vi "convert_string2list.vi"(0 "PARSED STRING":string, 2 "BEGIN (CHAR)":string, 3 "TERM (CHAR)":string, 4 "CLUSTER (CHAR)":string, 5 "SEPARATOR (CHAR)":string) -> (14 "LIST":string[](array[string]), 19 "ERROR OUT":errorcluster)   [LabVIEW 2018, in "db_lib R3.lvlib"]
uses:
  db_lib R3.lvlib
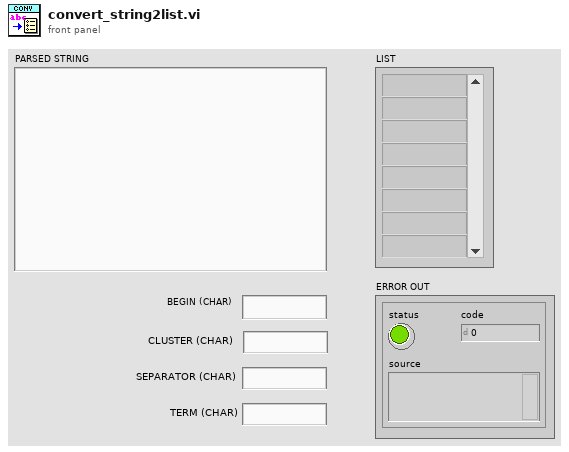
[diagram p1: front panel]
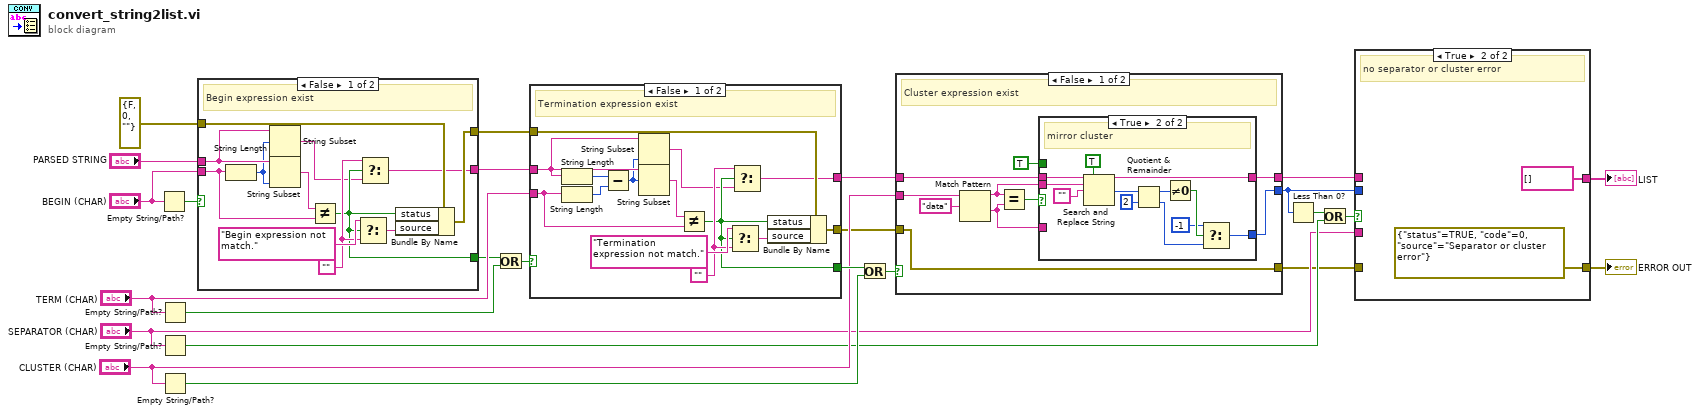
[diagram p0: block diagram]
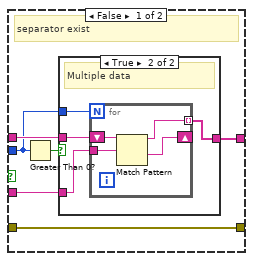
[diagram p2: hidden frame]
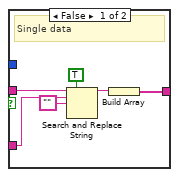
[diagram p3: hidden frame]
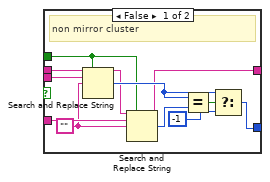
[diagram p4: hidden frame]
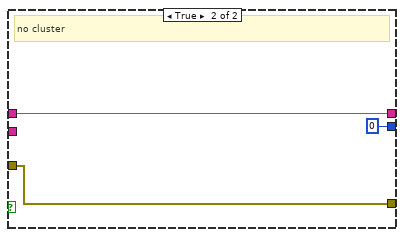
[diagram p5: hidden frame]
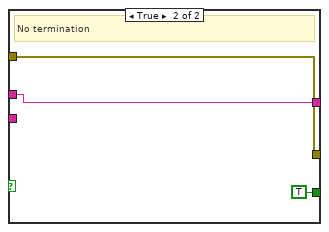
[diagram p6: hidden frame]
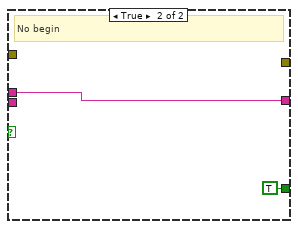
[diagram p7: hidden frame]
diagram:
  n1 = Empty String/Path?(string/path="BEGIN (CHAR)") -> (empty?=w25:bool)
  n2 = Empty String/Path?(string/path="TERM (CHAR)") -> (empty?=w16:bool)
  n3 = Empty String/Path?(string/path="SEPARATOR (CHAR)") -> (empty?=w7:bool)
  n4 = Empty String/Path?(string/path="CLUSTER (CHAR)") -> (empty?=w9:bool)
  n5 = case shown="False" w25 {
    tunnel: "PARSED STRING" -> [w34 w39]
    tunnel: [w30 w39] -> w21
    tunnel: "BEGIN (CHAR)" -> [w35 _]
    tunnel: errorcluster {"status"=FALSE, "code"=0, "source"=""} ("error constant") -> [w36 _]
    tunnel: [w31 _] -> w20
    tunnel: [w27 TRUE] -> w17
    frame False {
      w28 = ""
      # "Begin expression exist"
      n6 = String Length(string=w35) -> (length=w33:i32)
      n7 = String Subset(string=w34, offset (0)=w33) -> (substring=w26:string)  [unwired: 1 in]
      n8 = String Subset(string=w34, length (rest)=w33) -> (substring=w37:string)  [unwired: 1 in]
      n9 = Not Equal?(x=w37, y=w35) -> (x != y?=w27:bool)
      n10 = Select(t="Begin expression not match.", s=w27, f=w28) -> (s? t:f=w32:string)
      n11 = Select(t=w28, s=w27, f=w26) -> (s? t:f=w30:string)
      n12 = Bundle By Name(cluster=w36, "status"=w27, "source"=w32) -> (w31:errorcluster)
    }
    frame True {
      # "No begin"
    }
  }
  n13 = Or(x=w17, y=w16) -> (x .or. y?=w19:bool)
  n14 = case shown="False" w19 {
    tunnel: w21 -> [w46 w54]
    tunnel: [w49 w54] -> w14
    tunnel: "TERM (CHAR)" -> [w52 _]
    tunnel: w20 -> [w53 w56]
    tunnel: [w50 w56] -> w11
    tunnel: [w41 TRUE] -> w15
    frame False {
      w47 = ""
      # "Termination expression exist"
      n15 = String Length(string=w46) -> (length=w45:i32)
      n16 = String Length(string=w52) -> (length=w44:i32)
      n17 = Subtract(x=w45, y=w44) -> (x-y=w42:i32)
      n18 = String Subset(string=w46, length (rest)=w42) -> (substring=w40:string)  [unwired: 1 in]
      n19 = String Subset(string=w46, offset (0)=w42) -> (substring=w43:string)  [unwired: 1 in]
      n20 = Not Equal?(x=w43, y=w52) -> (x != y?=w41:bool)
      n21 = Select(t="Termination expression not match.", s=w41, f=w47) -> (s? t:f=w51:string)
      n22 = Select(t=w47, s=w41, f=w40) -> (s? t:f=w49:string)
      n23 = Bundle By Name(cluster=w53, "status"=w41, "source"=w51) -> (w50:errorcluster)
    }
    frame True {
      # "No termination"
    }
  }
  n24 = Or(x=w15, y=w9) -> (x .or. y?=w13:bool)
  n25 = case shown="False" w13 {
    tunnel: w14 -> [w63 w93]
    tunnel: "CLUSTER (CHAR)" -> [w66 _]
    tunnel: [w59 w93] -> w6
    tunnel: [w58 0 ("t")] -> w4
    tunnel: w11 -> [w57 w91]
    tunnel: [w57 w91] -> w2
    frame False {
      # "Cluster expression exist"
      n26 = Match Pattern(string=w66, regular expression="data") -> (before substring=w62:string, after substring=w61:string)  [unwired: 1 in, 2 out]
      n27 = Equal?(x=w62, y=w61) -> (x = y?=w64:bool)
      n28 = case shown="True" w64 {
        tunnel: w63 -> [w77 w90]
        tunnel: w62 -> [w78 w89]
        tunnel: [w68 w86] -> w59
        tunnel: w61 -> [w76 _]
        tunnel: [w71 w79] -> w58
        tunnel: TRUE -> [w67 _]
        frame False {
          w70 = ""
          # "non mirror cluster"
          n29 = Search and Replace String(replace all?=w67, input string=w77, search string=w78, replace string=w70) -> (result string=w69:string, number of replacements=w73:i32)  [unwired: 4 in, 2 out]
          n30 = Search and Replace String(replace all?=w67, input string=w69, search string=w76, replace string=w70) -> (result string=w68:string, number of replacements=w74:i32)  [unwired: 4 in, 2 out]
          n31 = Equal?(x=w73, y=w74) -> (x = y?=w75:bool)
          n32 = Select(t=w73, s=w75, f=-1) -> (s? t:f=w71:i32)
        }
        frame True {
          # "mirror cluster"
          n33 = Search and Replace String(replace all?=TRUE ("replace all? (F)"), input string=w90, search string=w89, replace string="") -> (result string=w86:string, number of replacements=w85:i32)  [unwired: 4 in, 2 out]
          n34 = Quotient & Remainder(x=w85, y=2) -> (x-y*floor(x/y)=w84:i32, floor(x/y)=w82:i32)
          n35 = Not Equal To 0?(x=w84) -> (x != 0?=w83:bool)
          n36 = Select(t=-1, s=w83, f=w82) -> (s? t:f=w79:i32)
        }
      }
    }
    frame True {
      # "no cluster"
    }
  }
  n37 = Less Than 0?(x=w4) -> (x < 0?=w10:bool)
  n38 = Or(x=w10, y=w7) -> (x .or. y?=w8:bool)
  n39 = case shown="True" w8 {
    tunnel: w6 -> [w98 _]
    tunnel: "SEPARATOR (CHAR)" -> [w97 _]
    tunnel: w4 -> [w95 _]
    tunnel: [w96 string[] []] -> w3
    tunnel: w2 -> [w94 _]
    tunnel: [w94 errorcluster {"status"=TRUE, "code"=0, "source"="Separator or cluster error"} ("error constant")] -> w1
    frame False {
      # "separator exist"
      n40 = Greater Than 0?(x=w95) -> (x > 0?=w99:bool)
      n41 = case shown="True" w99 {
        tunnel: w98 -> [w105 w108]
        tunnel: w97 -> [w104 w107]
        tunnel: [w100 w106] -> w96
        tunnel: w95 -> [_ w109]
        frame False {
          # "Single data"
          n42 = Search and Replace String(replace all?=TRUE ("replace all? (F)"), input string=w105, search string=w104, replace string="") -> (result string=w101:string)  [unwired: 4 in, 3 out]
          n43 = Build Array(w101) -> (w100:string[])
        }
        frame True {
          # "Multiple data"
          n44 = for {
            N: w109 -> [_]
            tunnel: w107 -> [w112]
            tunnel: [w111] -> w106 mode=indexing
            shift-right: [w110] -> _
            shift-left: w108 -> [w113]
            n45 = Match Pattern(string=w113, regular expression=w112) -> (before substring=w111:string, after substring=w110:string)  [unwired: 1 in, 2 out]
          }
        }
      }
    }
    frame True {
      # "no separator or cluster error"
    }
  }
  "LIST" <- w3
  "ERROR OUT" <- w1
